vi "JJMCclase2.vi"() -> ()   [LabVIEW 2011]
panel:
  out "Temperatura Agradable":bool
  out "Alarma":bool
  out "Valor Temperatura":dbl
  out "Temperatura":i32(slide) scale=0.0..60.0
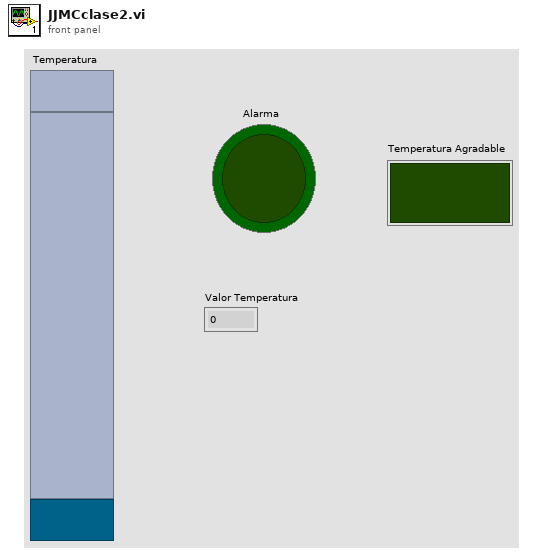
[diagram p1: front panel]
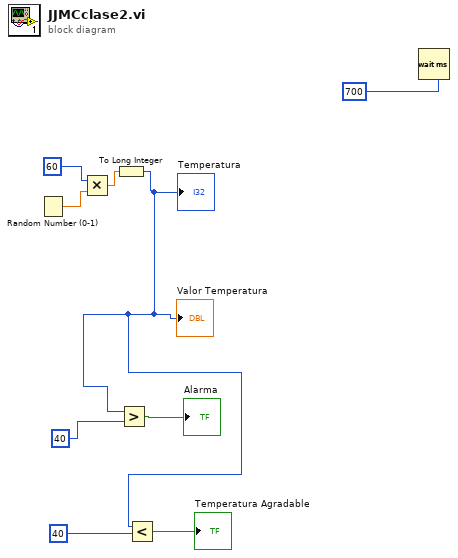
[diagram p0: block diagram]
diagram:
  n1 = Random Number (0-1)() -> (number: 0 to 1=w8:dbl)
  n2 = Multiply(x=60, y=w8) -> (x*y=w7:dbl)
  n3 = To Long Integer(number=w7) -> (32bit integer=w2:i32)
  "Temperatura" <- w2
  "Valor Temperatura" <- w2
  n4 = Greater?(x=w2, y=40) -> (0:→"Alarma":bool)
  n5 = Less?(x=w2, y=40) -> (x < y?=→"Temperatura Agradable":bool)
  n6 = Wait (ms)(milliseconds to wait=700) -> ()  [unwired: 1 out]
